vi "svx_Orbit Autoscale.vi"(6 "Display State In":T1={"X Scale"={"Name"="Horizontal", "FString"="%#.2g", "Major Color"=16777238, "Minor Color"=16777216, "Scale Visible"=TRUE, " Label Visible"=TRUE, "Grid Style"=1}, "Y Scale"={"Name"="Vertical", "FString"="%#.2g", "Major Color"=16777238, "Minor Color"=16777216, "Scale Visible"=TRUE, " Label Visible"=TRUE, "Grid Style"=1}, "Plot"={"Point Style"=0, "Line Width"=0, "Line Style"=0, "Plot Color"=9727, "Point/fill"=0}, "Arrow/Crosshair Color"=9727, "Tacho Point Color"=16711680, "Container Bounds"={"Width"=563, "Height"=294}, "Axis Maximum"=10.0, "Probe Angles"={"Angle X"=0.0, "Angle Y"=1.5707963267948966}, "Background Color"=16777226, "Cursor"={"Cursor Point Style"=13, "Cursor Style"=4, "Cursor Line Width"=1, "Cursor Line Style"=0, "Cursor Color"=9727, "Cursor Name Visible"=TRUE, "Cursor Visible"=TRUE, "Cursor Position"={"X"=0.0, "Y"=0.0}, "Cursor Index"=0, "Cursor Lock"=FALSE}, "Elliptical Info"=[], "Legend Visible"=TRUE, "Scale Range Change"=refnum, "Strings[]"={"Custom pair name"=FALSE, "Row Strings []"=[], "Column Strings []"=[]}, "Index"=[{"pair index"=0, "order index"=0}], " Parents Tags"=[], "Children Tags"=[], "Open?"=[], "Label"="", "Legend Width"=120, "Pair Strings Changed?"=FALSE, "Size"=[], "Legend Background"=16777226, "Legend Font"=16777222, "Cursor Release"=refnum, "Autoscale"=TRUE, "Precession Direction"=[], "Item Width"=0, "User Pair Strings []"=[], "Users Order Strings []"=[], "Autoscale Once"=TRUE, "Property Write"=refnum} caption="State" {"Index"."order index" min=0; "Index"."pair index" min=0; "Axis Maximum" min=0.0}, 7 "Orbit Plot":T3, 11 "Orbit Plot":refnum<vi>) -> (4 "Display State Out":T1={"X Scale"={"Name"="Horizontal", "FString"="%#.2g", "Major Color"=16777238, "Minor Color"=16777216, "Scale Visible"=TRUE, " Label Visible"=TRUE, "Grid Style"=1}, "Y Scale"={"Name"="Vertical", "FString"="%#.2g", "Major Color"=16777238, "Minor Color"=16777216, "Scale Visible"=TRUE, " Label Visible"=TRUE, "Grid Style"=1}, "Plot"={"Point Style"=0, "Line Width"=0, "Line Style"=0, "Plot Color"=9727, "Point/fill"=0}, "Arrow/Crosshair Color"=9727, "Tacho Point Color"=16711680, "Container Bounds"={"Width"=563, "Height"=294}, "Axis Maximum"=10.0, "Probe Angles"={"Angle X"=0.0, "Angle Y"=1.5707963267948966}, "Background Color"=16777226, "Cursor"={"Cursor Point Style"=13, "Cursor Style"=4, "Cursor Line Width"=1, "Cursor Line Style"=0, "Cursor Color"=9727, "Cursor Name Visible"=TRUE, "Cursor Visible"=TRUE, "Cursor Position"={"X"=0.0, "Y"=0.0}, "Cursor Index"=0, "Cursor Lock"=FALSE}, "Elliptical Info"=[], "Legend Visible"=TRUE, "Scale Range Change"=refnum, "Strings[]"={"Custom pair name"=FALSE, "Row Strings []"=[], "Column Strings []"=[]}, "Index"=[{"pair index"=0, "order index"=0}], " Parents Tags"=[], "Children Tags"=[], "Open?"=[], "Label"="", "Legend Width"=120, "Pair Strings Changed?"=FALSE, "Size"=[], "Legend Background"=16777226, "Legend Font"=16777222, "Cursor Release"=refnum, "Autoscale"=TRUE, "Precession Direction"=[], "Item Width"=0, "User Pair Strings []"=[], "Users Order Strings []"=[], "Autoscale Once"=TRUE, "Property Write"=refnum} caption="State" {"Index"."order index" min=0; "Index"."pair index" min=0; "Axis Maximum" min=0.0})   [LabVIEW 2017, in "SVX Orbit.xctl"]
uses:
  <vilib>/addons/_XControls/Orbit Plot/SVX Orbit.xctl
  <vilib>/addons/_XControls/Orbit Plot/subVIs/svx_Orbit Internal State.ctl
  <vilib>/addons/_XControls/Orbit Plot/subVIs/svx_Orbit Bounds.ctl
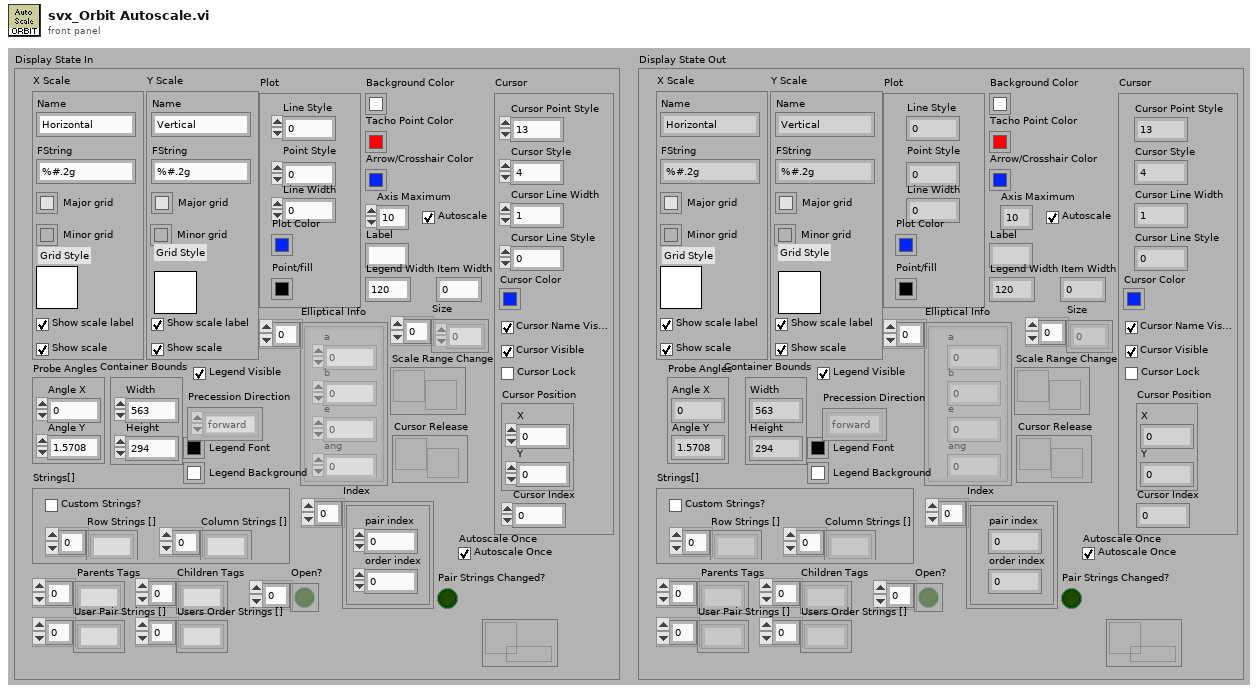
[diagram p1: front panel]
types:
  T1 = typedef "SVX Orbit.xctl/svx_Orbit Internal State.ctl" = cluster{"X Scale":cluster{"Name":string, "FString":string, "Major Color":u32, "Minor Color":u32, "Scale Visible":bool, " Label Visible":bool, "Grid Style":u16}, "Y Scale":cluster{"Name":string, "FString":string, "Major Color":u32, "Minor Color":u32, "Scale Visible":bool, " Label Visible":bool, "Grid Style":u16}, "Plot":cluster{"Point Style":u8, "Line Width":u8, "Line Style":u8, "Plot Color":u32, "Point/fill":u32}, "Arrow/Crosshair Color":u32, "Tacho Point Color":u32, "Container Bounds":T2, "Axis Maximum":dbl, "Probe Angles":cluster{"Angle X":dbl, "Angle Y":dbl}, "Background Color":u32, "Cursor":cluster{"Cursor Point Style":u8, "Cursor Style":u8, "Cursor Line Width":u8, "Cursor Line Style":u8, "Cursor Color":u32, "Cursor Name Visible":bool, "Cursor Visible":bool, "Cursor Position":cluster{"X":dbl, "Y":dbl}, "Cursor Index":i32, "Cursor Lock":bool}, "Elliptical Info":cluster{"a":dbl, "b":dbl, "e":dbl, "ang":dbl}[], "Legend Visible":bool, "Scale Range Change":refnum<user-event>, "Strings[]":cluster{"Custom pair name":bool, "Row Strings []":string[], "Column Strings []":string[]}, "Index":cluster{"pair index":i32, "order index":i32}[], " Parents Tags":string[], "Children Tags":string[], "Open?":bool[], "Label":string, "Legend Width":u32, "Pair Strings Changed?":bool, "Size":i32[], "Legend Background":u32, "Legend Font":u32, "Cursor Release":refnum<user-event>, "Autoscale":bool, "Precession Direction":enum16{"forward", "backward"}[], "Item Width":u32, "User Pair Strings []":string[], "Users Order Strings []":string[], "Autoscale Once":bool, "Property Write":refnum<queue>}
  T2 = typedef "SVX Orbit.xctl/svx_Orbit Bounds.ctl" = cluster{"Width":u32, "Height":u32}
  T3 = cluster{"X":dbl[], "Y":dbl[], "reference":dbl[], "plot type":enum16{"Filtered Plot", "Unfiltered Plot"}, "attribute":variant}
  T4 = cluster{"orbit plot X":dbl[], "orbit plot Y":dbl[]}[]
  T5 = cluster{"orbit plot X":dbl[], "orbit plot Y":dbl[]}
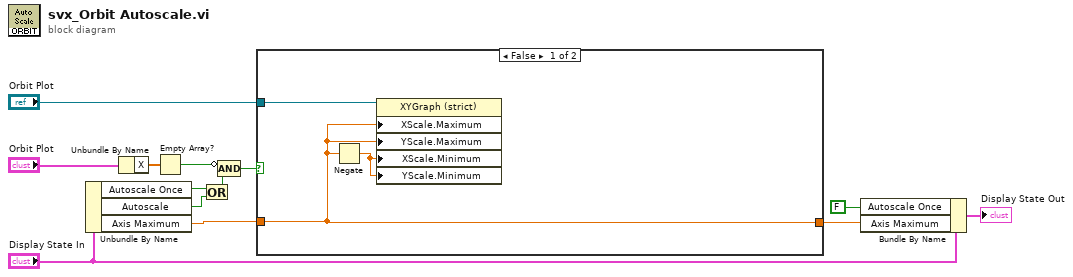
[diagram p0: block diagram]
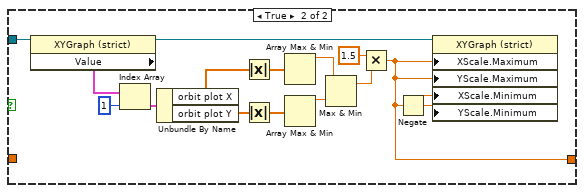
[diagram p2: hidden frame]
diagram:
  n1 = Unbundle By Name("Display State In") -> ("Autoscale Once"=w10:bool, "Autoscale"=w9:bool, "Axis Maximum"=w2:dbl)
  n2 = Unbundle By Name("Orbit Plot") -> ("X"=w12:dbl[])
  n3 = Empty Array?(array=w12) -> (empty?=w7:bool)
  n4 = Or(x=w10, y=w9) -> (x .or. y?=w8:bool)
  n5 = Compound Arithmetic op=AND(invert w7, w8) -> (w6:bool)
  n6 = case shown="False" w6 {
    tunnel: "Orbit Plot" -> [w15 w28]
    tunnel: [w14 w17] -> w3
    tunnel: w2 -> [w14 _]
    frame False {
      n7 = Negate(x=w14) -> (-x=w16:dbl)
      n8 = property on="Property Node" class="XYGraph (strict)"(reference=w15, "XScale.Maximum"=w14, "YScale.Maximum"=w14, "XScale.Minimum"=w16, "YScale.Minimum"=w16) -> ()  [unwired: 1 in, 2 out]
    }
    frame True {
      n9 = property on="Property Node" class="XYGraph (strict)"(reference=w28) -> (reference out=w26:refnum<vi>, "Value"=w31:T4)  [unwired: 1 in, 1 out]
      n10 = Index Array(array=w31, index=1) -> (element=w30:T5)
      n11 = Unbundle By Name(w30) -> ("orbit plot X"=w23:dbl[], "orbit plot Y"=w25:dbl[])
      n12 = Absolute Value(x=w23) -> (abs(x)=w22:dbl[])
      n13 = Absolute Value(x=w25) -> (abs(x)=w24:dbl[])
      n14 = Array Max & Min(array=w22) -> (max value=w27:dbl)  [unwired: 3 out]
      n15 = Array Max & Min(array=w24) -> (max value=w29:dbl)  [unwired: 3 out]
      n16 = Max & Min(x=w27, y=w29) -> (max(x,y)=w20:dbl)  [unwired: 1 out]
      n17 = Multiply(x=1.5, y=w20) -> (x*y=w17:dbl)
      n18 = Negate(x=w17) -> (-x=w21:dbl)
      n19 = property on="Property Node" class="XYGraph (strict)"(reference=w26, "XScale.Maximum"=w17, "YScale.Maximum"=w17, "XScale.Minimum"=w21, "YScale.Minimum"=w21) -> ()  [unwired: 1 in, 2 out]
    }
  }
  n20 = Bundle By Name(cluster="Display State In", "Autoscale Once"=FALSE, "Axis Maximum"=w3) -> (→"Display State Out":T1)
